vi "Usage Buttons.vi"() -> ()   [LabVIEW 2011, in "Wiimote.lvlib"]
uses:
  Wiimote.lvlib
  Wiimote Buttons.ctl
panel:
  in  "index":i32
  out "Wiimote Buttons out":T1
  in  "stop":bool
  out "error out":errorcluster
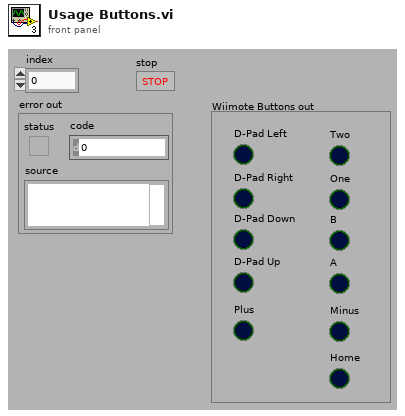
[diagram p1: front panel]
types:
  T1 = typedef "Wiimote.lvlib/Wiimote Buttons.ctl" = cluster{"D-Pad Left":bool, "D-Pad Right":bool, "D-Pad Down":bool, "D-Pad Up":bool, "Plus":bool, "Two":bool, "One":bool, "B":bool, "A":bool, "Minus":bool, "Home":bool}
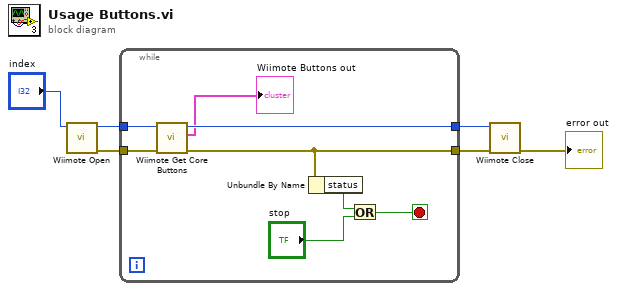
[diagram p0: block diagram]
diagram:
  n1 = call "Wiimote Open.vi"("index"="index") -> ("error out"=w1:errorcluster, "hWiimoteHandle"=w2:u32)  [unwired: 9 in]
  n2 = while {
    tunnel: [w13] -> w5
    tunnel: [w14] -> w4
    tunnel: w2 -> [w9]
    tunnel: w1 -> [w8]
    stop <- w11 stop-if-true
    n3 = call "Wiimote Get Core Buttons.vi"("error in"=w8, "hWiimoteHandle in"=w9) -> ("error out"=w13:errorcluster, "Wiimote Buttons out"=→"Wiimote Buttons out":T1, "hWiimoteHandle out"=w14:u32)  [unwired: 7 in]
    n4 = Unbundle By Name(w13) -> ("status"=w12:bool)
    n5 = Or(x=w12, y="stop") -> (x .or. y?=w11:bool)
  }
  n6 = call "Wiimote Close.vi"("error in"=w5, "hWiimoteHandle in"=w4) -> ("error out"=→"error out":errorcluster)  [unwired: 9 in]
